vi "IO_Switch_#1(S1).vi"(8 "error in":errorcluster, 10 "Output":T1(ring)=enum."AHR (J2)", 11 "Input":T2(ring)=enum."Splitter") -> (0 "error out":errorcluster, 2 "Verfied":bool, 3 "Switches":string)   [LabVIEW 2012]
panel:
  # "IO Switch #1 (S1)"
  # "Switch Output"
  # "Switch Input"
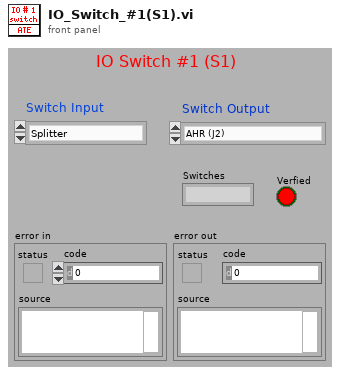
[diagram p1: front panel]
types:
  T1 = enum16{"NONE", "AHR (J2)", "Delay Device (S4)", "Power Meter Switch (S5)", "Reversing Switch"}
  T2 = enum16{"NONE", "AHR (J2)", "Splitter", "Signal Out Switch (S3)", "Reversing Switch", "Power Meter Switch"}
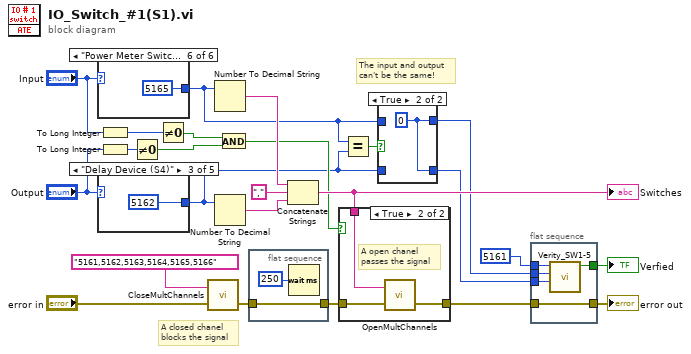
[diagram p0: block diagram]
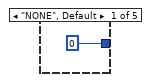
[diagram p3: hidden frame]
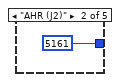
[diagram p4: hidden frame]
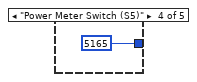
[diagram p5: hidden frame]
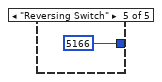
[diagram p6: hidden frame]
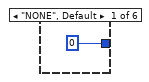
[diagram p7: hidden frame]
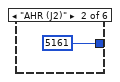
[diagram p8: hidden frame]
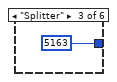
[diagram p9: hidden frame]
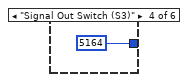
[diagram p10: hidden frame]
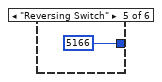
[diagram p11: hidden frame]
diagram:
  # "The input and output\ncan't be the same!"
  # "A closed chanel\nblocks the signal"
  n1 = case shown="\"Power Meter Switch\"" "Input" {
    tunnel: [0 ("Switch ID") 5161 ("Switch ID") 5163 ("Switch ID") 5164 ("Switch ID") 5166 ("Switch ID") 5165 ("Switch ID")] -> w2
    frame "NONE", Default {
    }
    frame "AHR (J2)" {
    }
    frame "Splitter" {
    }
    frame "Signal Out Switch (S3)" {
    }
    frame "Reversing Switch" {
    }
    frame "Power Meter Switch" {
    }
  }
  n2 = case shown="\"Delay Device (S4)\"" "Output" {
    tunnel: [0 ("Switch ID") 5161 ("Switch ID") 5162 ("Switch ID") 5165 ("Switch ID") 5166 ("Switch ID")] -> w4
    frame "NONE", Default {
    }
    frame "AHR (J2)" {
    }
    frame "Delay Device (S4)" {
    }
    frame "Power Meter Switch (S5)" {
    }
    frame "Reversing Switch" {
    }
  }
  n3 = To Long Integer(number="Input") -> (32bit integer=w14:i32)
  n4 = To Long Integer(number="Output") -> (32bit integer=w13:i32)
  n5 = Not Equal To 0?(x=w13) -> (x != 0?=w12:bool)
  n6 = Not Equal To 0?(x=w14) -> (x != 0?=w11:bool)
  n7 = call "CloseMultChannels.vi"("error in (no error)"="error in", "Channels to be closed"="5161,5162,5163,5164,5165,5166" ("Channels to be opened")) -> ("error out"=w20:errorcluster)  [unwired: 1 in]
  n8 = Number To Decimal String(number=w2) -> (decimal integer string=w17:string)  [unwired: 1 in]
  n9 = Number To Decimal String(number=w4) -> (decimal integer string=w18:string)  [unwired: 1 in]
  n10 = And(x=w11, y=w12) -> (x .and. y?=w10:bool)
  n11 = flat-sequence {
    tunnel: w20 -> [w36]
    tunnel: [w36] -> w19
    frame #0 {
      n12 = Wait (ms)(milliseconds to wait=u32 250) -> ()  [unwired: 1 out]
    }
  }
  n13 = Concatenate Strings(w17, ",", w18) -> (w21:string)
  "Switches" <- w21
  n14 = case shown="True" w10 {
    tunnel: w19 -> [w38 w40]
    tunnel: w21 -> [_ w41]
    tunnel: [w38 w39] -> w9
    frame False {
    }
    frame True {
      # "A open chanel\npasses the signal"
      n15 = call "OpenMultChannels.vi"("error in (no error)"=w40, "Channels to be opened"=w41) -> ("error out"=w39:errorcluster)  [unwired: 1 in]
    }
  }
  n16 = Equal?(x=w2, y=w4) -> (x = y?=w5:bool)
  n17 = case shown="True" w5 {
    tunnel: w4 -> [w42 _]
    tunnel: [w42 w44] -> w3
    tunnel: w2 -> [w43 _]
    tunnel: [w43 w44] -> w1
    frame False {
    }
    frame True {
      w44 = 0 ("Switch ID")
    }
  }
  n18 = flat-sequence {
    tunnel: 5161 ("Switch ID") -> [w49]
    tunnel: w1 -> [w48]
    tunnel: w3 -> [w47]
    tunnel: [w46] -> w6
    tunnel: w9 -> [w45]
    tunnel: [w45] -> w8
    frame #0 {
      n19 = call "Verity_SW1-5.vi"("Output Switch ID"=w47, "Input Switch ID"=w48, "Base Switch ID"=w49) -> ("Verfied"=w46:bool)  [unwired: 7 in, 1 out]
    }
  }
  "error out" <- w8
  "Verfied" <- w6
